vi "LVClass_Pupil Read Pupil.vi"(8 "error in (no error)":errorcluster, 11 "Pupil in":refnum<class "Pupil.lvclass">) -> (0 "error out":errorcluster, 2 "Pupil":T1, 3 "Pupil out":refnum<class "Pupil.lvclass">)   [LabVIEW 2020, in "Pupil.lvclass"]
uses:
  Pupil.lvclass
  ClassID.ctl
  Pupil.lvclass/Pupil.ctl
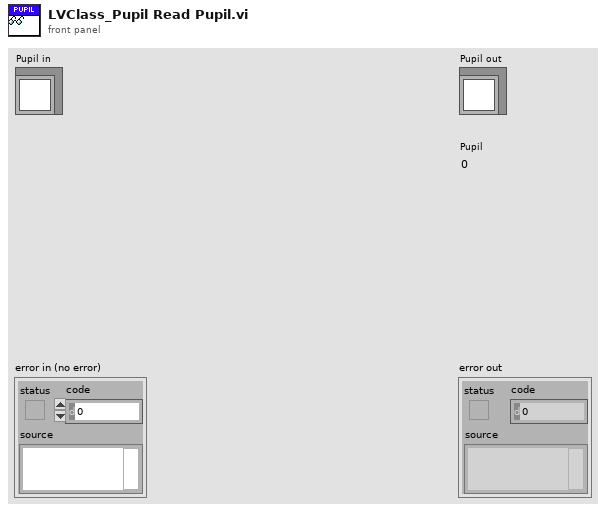
[diagram p1: front panel]
types:
  T1 = typedef "ClassID.ctl" = i64
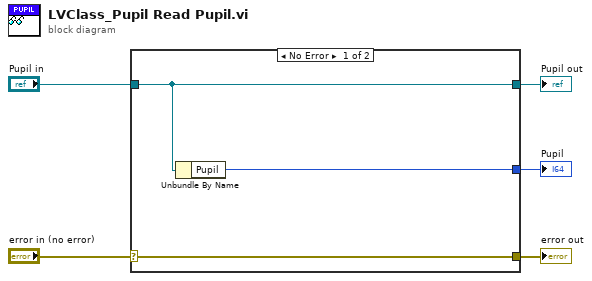
[diagram p0: block diagram]
diagram:
  n1 = case shown="No Error" "error in (no error)" {
    selector: "error in (no error)" -> [w8 w9]
    tunnel: [w8 w9] -> w4
    tunnel: [w7 w10] -> w2
    tunnel: "Pupil in" -> [w7 w10]
    tunnel: [w6 _] -> w1
    frame No Error {
      n2 = Unbundle By Name(w7) -> ("Pupil"=w6:T1)
    }
    frame Error {
    }
  }
  "error out" <- w4
  "Pupil out" <- w2
  "Pupil" <- w1
